vi "总磷单步调试对话框.vi"() -> ()   [LabVIEW 2016, in "斯坦道总氮V2.lvlib"]
panel:
  in  "单步调试":T8={"注射泵"=enum."注入", "阀口选择"=enum."V1", "灯"=enum."未选择", "ADC值"=enum."未选择", "数值"=4000, "项目输入"=0, "控温"=enum."未选择", "外设选择"=enum."未选择", "外设选择2"={"V9-1"=FALSE, "V9-2"=FALSE}} {"项目输入" items=["总磷"=1, "总氮"=2, "氨氮"=3, "磷酸盐"=4, "硝氮"=5, "亚硝氮"=6, "硅酸盐"=7, "硫化物"=8, "CODcr"=22, "氟化物"=50]}
  in  "停止":bool
  out "注射器温度":sgl
  out "消解温度":sgl
  out "ADC":sgl
  out "F3":sgl format="%#.6f"
  out "F2":sgl format="%#.6f"
  out "F1":sgl format="%#.6f"
  out "F0":sgl format="%#.6f"
  in  "退出":bool
  in  "启动":bool
  # "单步调试界面"
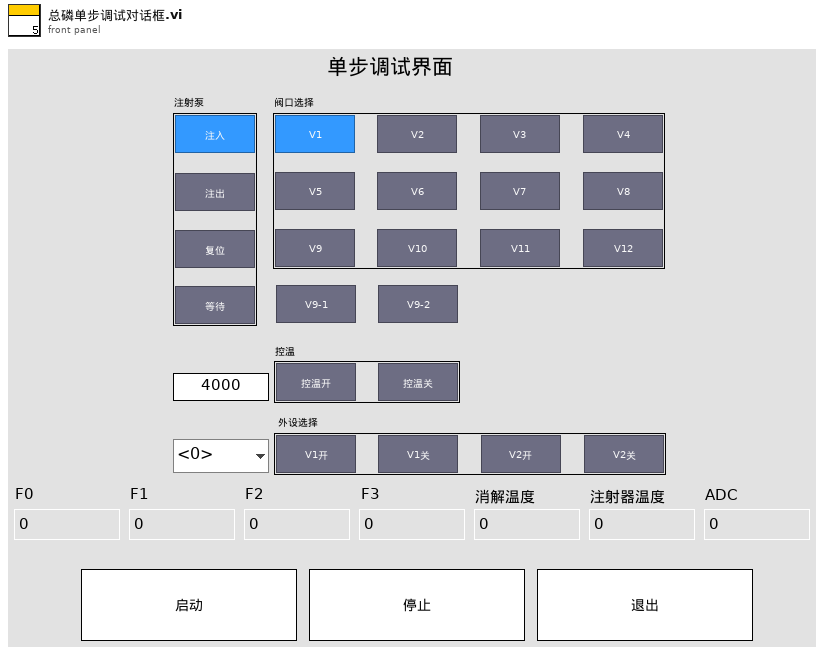
[diagram p1: front panel]
types:
  T1 = typedef "SingleStepTestV2.lvlib/SingleStepTestV2.lvclass/注射泵操作.ctl" = enum32{"复位", "注入", "注出", "等待"}
  T2 = typedef "SingleStepTestV2.lvlib/SingleStepTestV2.lvclass/阀口操作.ctl" = enum32{"未选择", "V1", "V2", "V3", "V4", "V5", "V6", "V7", "V8", "V9", "V10", "V11", "V12"}
  T3 = typedef "SingleStepTestV2.lvlib/SingleStepTestV2.lvclass/灯选择.ctl" = enum32{"未选择", "520", "660", "加热恒温", "氙灯/紫灯"}
  T4 = typedef "SingleStepTestV2.lvlib/SingleStepTestV2.lvclass/ADC选择.ctl" = enum32{"未选择", "ADC0", "降温温度", "消解温度", "光谱/ADC1"}
  T5 = typedef "SingleStepTestV2.lvlib/SingleStepTestV2.lvclass/控温操作.ctl" = enum32{"未选择", "控温开", "控温关"}
  T6 = typedef "SingleStepTestV2.lvlib/SingleStepTestV2.lvclass/外设选择.ctl" = enum32{"未选择", "V1开", "V1关", "V2开", "V2关"}
  T7 = typedef "SingleStepTestV2.lvlib/SingleStepTestV2.lvclass/外设选择2.ctl" = cluster{"V9-1":bool, "V9-2":bool}
  T8 = cluster{"注射泵":T1, "阀口选择":T2, "灯":T3, "ADC值":T4, "数值":i16, "项目输入":u16, "控温":T5, "外设选择":T6, "外设选择2":T7}
  T9 = cluster{"时间标识":timestamp, "设备":string, "日志信息":string, "流程参数":string}
  T10 = cluster{"系统时间":timestamp, "工作状态":u16, "测量模式":enum16{"待机", "连续模式", "周期模式", "定点模式", "受控模式", "手动模式"}, "告警代码":u16, "故障代码":u16, "日志代码":u16, "软件版本":u16, "F0":sgl, "F1":sgl, "F2":sgl, "F3":sgl, "T":sgl, "H":sgl, "id":u16, "flowid":u16, "量程":u16, "总磷控温温度1":sgl, "营养盐控温温度2":sgl, "ADC":sgl}
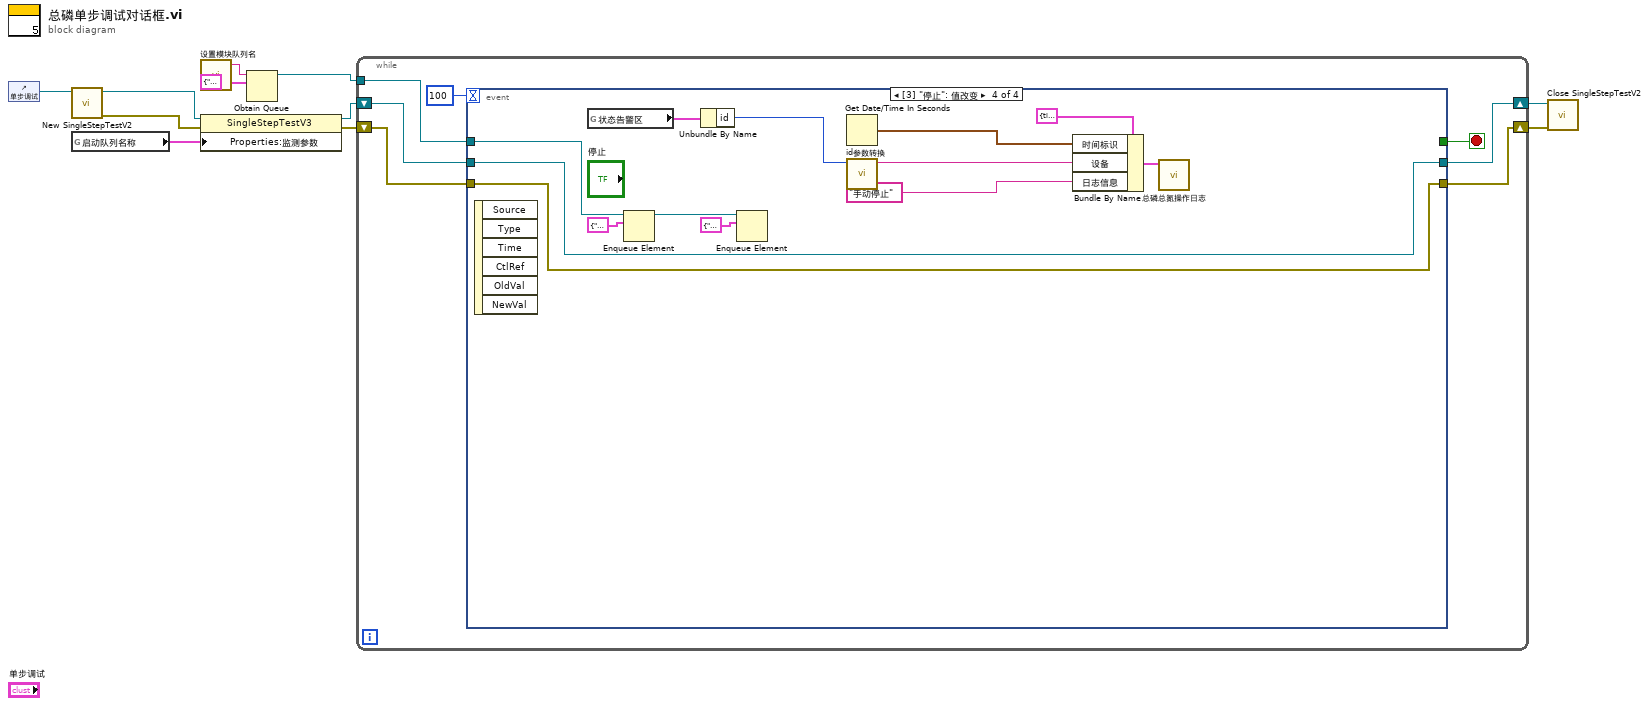
[diagram p0: block diagram]
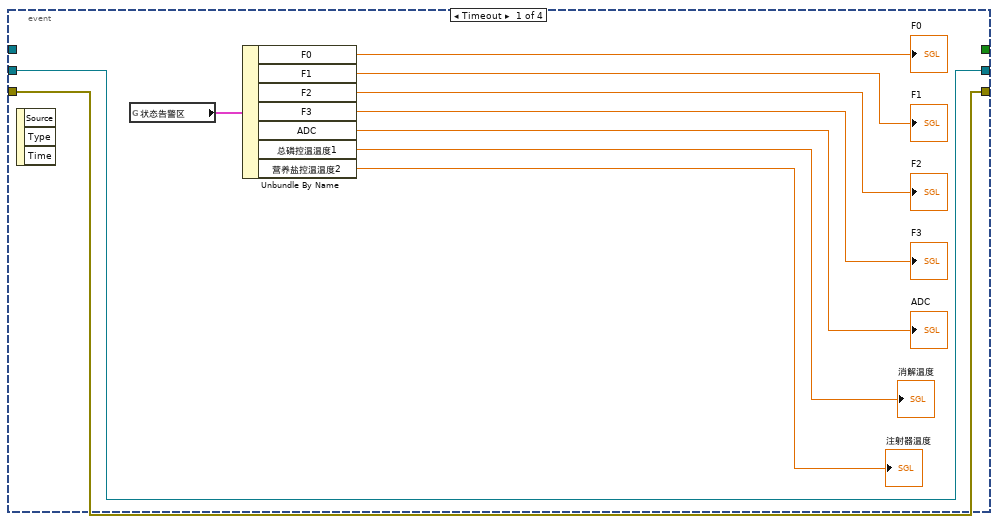
[diagram p2: hidden frame]
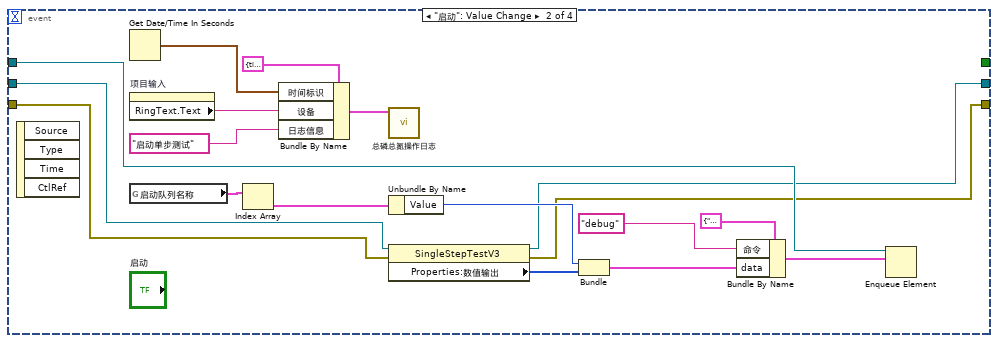
[diagram p3: hidden frame]
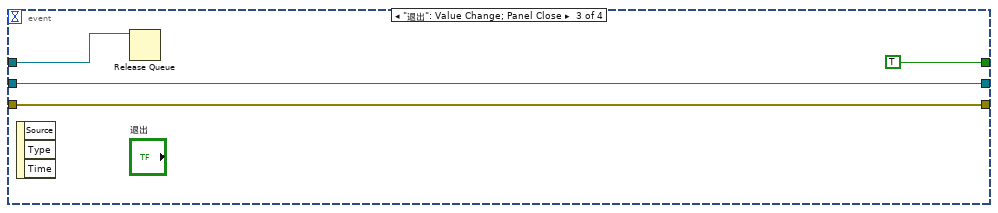
[diagram p4: hidden frame]
diagram:
  n1 = control-ref of="单步调试"() -> (w7:refnum<vi>)
  n2 = call "New SingleStepTestV2.vi"("Reference"=w7) -> ("error out"=w8:errorcluster, "SingleStepTestV3 out"=w2:refnum<class "SingleStepTestV2.lvclass">)  [unwired: 9 in]
  n3 = global read "总磷总氮断电保存全局变量.vi" "启动队列名称"() -> (w1:cluster{"String":string, "Value":u16}[])
  n4 = call "设置模块队列名.vi"() -> ("Msg"=w9:string)  [unwired: 5 in]
  n5 = property class="SingleStepTestV3"(reference=w2, error in=w8, "Properties:监测参数"=w1) -> (reference out=w6:refnum<class "SingleStepTestV2.lvclass">, error out=w5:errorcluster)
  n6 = Obtain Queue(name (unnamed)=w9, element data type=cluster{"命令":string, "data":variant} {"命令"="", "data"=variant}) -> (queue out=w10:refnum<queue>)  [unwired: 3 in, 2 out]
  n7 = while {
    tunnel: w10 -> [w18]
    shift-right: [w13] -> w4
    shift-left: w6 -> [w15]
    shift-right: [w12] -> w3
    shift-left: w5 -> [w14]
    stop <- w17 stop-if-true
    n8 = event shown="[3] \"停止\": 值改变" {
      selector: _ -> [_ _ _ _]
      dyn-events: _ -> [_ _ _ _]
      timeout: 100 -> [_ _ _ _]
      tunnel: w18 -> [_ w42 w49 w60]
      tunnel: [_ _ TRUE _] -> w17
      tunnel: w15 -> [w20 w38 w48 w59]
      tunnel: w14 -> [w19 w37 w47 w58]
      tunnel: [w20 w34 w48 w59] -> w13
      tunnel: [w19 w36 w47 w58] -> w12
      event Timeout {
        n9 = event-data() -> ()  [unwired: 1 in, 3 out]
        n10 = global read "VAR总磷总氮全局变量.vi" "状态告警区"() -> (w21:T10)
        n11 = Unbundle By Name(w21) -> ("F0"=→"F0":sgl, "F1"=→"F1":sgl, "F2"=→"F2":sgl, "F3"=→"F3":sgl, "ADC"=→"ADC":sgl, "总磷控温温度1"=→"消解温度":sgl, "营养盐控温温度2"=→"注射器温度":sgl)
      }
      event "启动": Value Change {
        n12 = event-data() -> ()  [unwired: 1 in, 4 out]
        n13 = Get Date/Time In Seconds() -> (seconds since 1Jan1904=w32:timestamp)
        n14 = property on="项目输入" class="Ring (严格)"() -> ("RingText.Text"=w29:string)  [unwired: 2 in, 2 out]
        n15 = global read "总磷总氮断电保存全局变量.vi" "启动队列名称"() -> (w39:cluster{"String":string, "Value":u16}[])
        n16 = Index Array(array=w39) -> (element=w41:cluster{"String":string, "Value":u16})  [unwired: 1 in]
        n17 = Bundle By Name(cluster=T9 {"时间标识"=timestamp(0 s since 1904-01-01), "设备"="", "日志信息"="", "流程参数"=""} ("data in"), "时间标识"=w32, "设备"=w29, "日志信息"="启动单步测试") -> (w31:T9)
        n18 = call "总磷总氮操作日志.vi"("data in"=w31) -> ()  [unwired: 10 in, 1 out]
        n19 = Unbundle By Name(w41) -> ("Value"=w40:u16)
        n20 = property class="SingleStepTestV3"(reference=w38, error in=w37) -> (reference out=w34:refnum<class "SingleStepTestV2.lvclass">, error out=w36:errorcluster, "Properties:数值输出"=w35:u16[])
        n21 = Bundle("Value"=w40, "Properties:数值输出"=w35) -> (w43:cluster{"Value":u16, "Properties:数值输出":u16[]})  [unwired: 1 in]
        n22 = Bundle By Name(cluster=cluster{"命令":string, "data":variant} {"命令"="", "data"=variant} ("元素"), "命令"="debug", "data"=w43) -> (w44:cluster{"命令":string, "data":variant})
        n23 = Enqueue Element(queue=w42, element=w44) -> ()  [unwired: 2 in, 3 out]
      }
      event "退出": Value Change; Panel Close {
        n24 = event-data() -> ()  [unwired: 1 in, 3 out]
        n25 = Release Queue(queue=w49) -> ()  [unwired: 2 in, 3 out]
      }
      event "停止": Value Change {
        n26 = event-data() -> ()  [unwired: 1 in, 6 out]
        n27 = global read "VAR总磷总氮全局变量.vi" "状态告警区"() -> (w53:T10)
        n28 = Enqueue Element(queue=w60, element=cluster{"命令":string, "data":variant} {"命令"="启动", "data"=variant(cluster{"站号":u16, "控制命令输出":u16[]} {"站号"=1, "控制命令输出"=[2816]})} ("元素")) -> (queue out=w61:refnum<queue>)  [unwired: 2 in, 2 out]
        n29 = Unbundle By Name(w53) -> ("id"=w52:u16)
        n30 = Enqueue Element(queue=w61, element=cluster{"命令":string, "data":variant} {"命令"="启动", "data"=variant(cluster{"站号":u16, "控制命令输出":u16[]} {"站号"=2, "控制命令输出"=[2816]})} ("元素")) -> ()  [unwired: 2 in, 3 out]
        n31 = Get Date/Time In Seconds() -> (seconds since 1Jan1904=w56:timestamp)
        n32 = call "id参数转换.vi"("id"=w52) -> ("table输出"=w51:string)  [unwired: 9 in, 1 out]
        n33 = Bundle By Name(cluster=T9 {"时间标识"=timestamp(0 s since 1904-01-01), "设备"="", "日志信息"="", "流程参数"=""} ("data in"), "时间标识"=w56, "设备"=w51, "日志信息"="手动停止") -> (w55:T9)
        n34 = call "总磷总氮操作日志.vi"("data in"=w55) -> ()  [unwired: 10 in, 1 out]
      }
    }
  }
  n35 = call "Close SingleStepTestV2.vi"("error in (no error)"=w3, "SingleStepTestV3 in"=w4) -> ()  [unwired: 9 in, 1 out]
